vi "measurement status.vi"(8 "error in (no error)":errorcluster, 10 "position":u16, 11 "busy":u16) -> (0 "error out":errorcluster, 2 "position out":u16, 3 "busy out":u16)   [LabVIEW 2015, in "SCANalone4x64.lvlib"]
doc: "__declspec(dllimport) void __stdcall measurement_status(unsigned short *busy, unsigned short *position);"
uses:
  <userlib>/SCANalone4x64/SCANalone4x64.lvlib
  <userlib>/SCANalone4x64/SCANalone4x64.dll
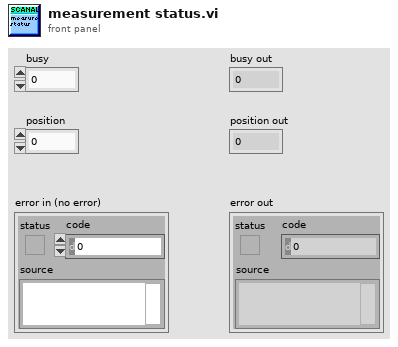
[diagram p1: front panel]
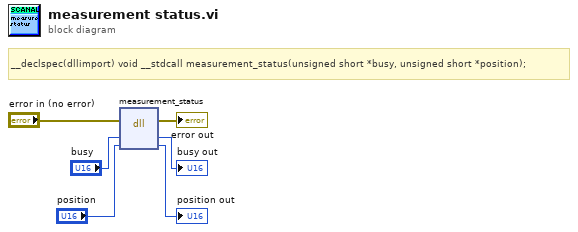
[diagram p0: block diagram]
diagram:
  # "__declspec(dllimport) void __stdcall measurement_status(unsigned short *busy, unsigned short *position);"
  n1 = dll-call lib="C:/Program Files/National Instruments/LabVIEW 2015/user.lib/SCANalone4x64/SCANalone4x64.*" fn="measurement_status"(error in="error in (no error)", "busy"="busy", "position"="position") -> (error out=→"error out":errorcluster, "busy"=→"busy out":u16, "position"=→"position out":u16)  [unwired: 3 in, 1 out]
